vi "VariantToData.vi"(1 "Variant":variant) -> (0 "Data":string[][](table))   [LabVIEW 2011]
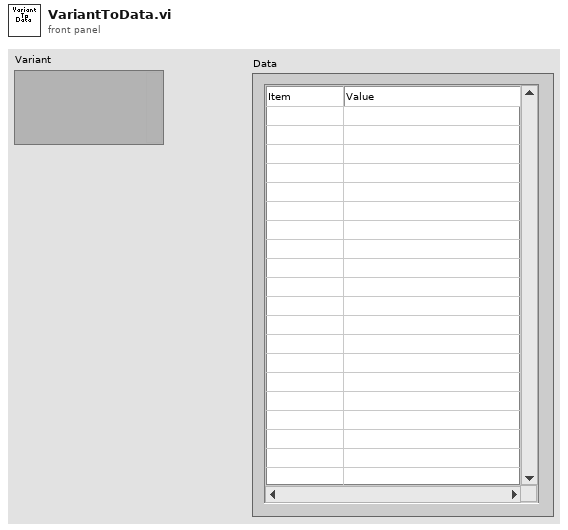
[diagram p1: front panel]
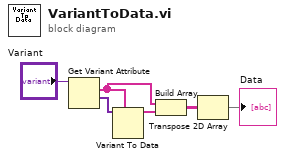
[diagram p0: block diagram]
diagram:
  n1 = Get Variant Attribute(Variant="Variant") -> (names=w3:string[], values=w5:variant[])  [unwired: 3 in, 2 out]
  n2 = Variant To Data(type=w3, Variant=w5) -> (data=w4:string[])  [unwired: 1 in, 1 out]
  n3 = Build Array(w3, w4) -> (w2:string[][])
  n4 = Transpose 2D Array(2D array=w2) -> (transposed array=→"Data":string[][])
